vi "ENA_statuses.vi"(8 "error in (no error)":errorcluster caption="错误输入（无错误）", 11 "MotorSystem 输入":refnum<class "MotorSystem.lvclass">) -> (0 "error out":errorcluster caption="错误输出", 2 "ENA statuses":bool[](array[boolean]), 3 "MotorSystem 输出":refnum<class "MotorSystem.lvclass">)   [LabVIEW 2016, in "MotionControl_UFO_3DOF.lvlib" / "MotorSystem.lvclass"]
uses:
  <userlib>/MotionControl_UFO_3DOF/MotorSystem/MotorSystem.lvclass
  <userlib>/MotionControl_UFO_3DOF/MotorSystem/MotorSystem.lvclass/MotorSystem.ctl
  <userlib>/MotionControl_UFO_3DOF/OneMotion/OneMotion.lvclass/OneMotion.ctl
  <userlib>/MotionControl_UFO_3DOF/StepMotor/StepMotor.lvclass
  <userlib>/MotionControl_UFO_3DOF/OneMotion/OneMotion.lvclass
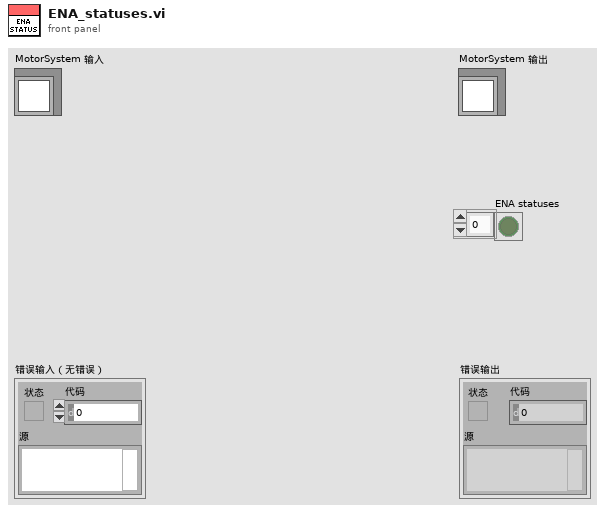
[diagram p1: front panel]
types:
  T1 = typedef "MotionControl_UFO_3DOF.lvlib/MotorSystem.lvclass/MotionCluster.ctl" = cluster{"OneMotion.lvclass":refnum<class "OneMotion.lvclass">, "connected?":bool, "default enabled?":bool, "enabled?":bool}
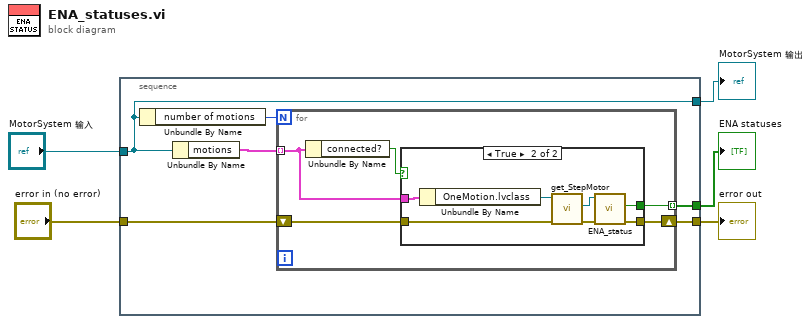
[diagram p0: block diagram]
diagram:
  n1 = stacked-sequence {
    tunnel: [w6] -> w5
    tunnel: [w11] -> w3
    tunnel: "MotorSystem 输入" -> [w11]
    tunnel: "error in (no error)" -> [w7]
    tunnel: [w8] -> w1
    frame #0 {
      n2 = Unbundle By Name(w11) -> ("number of motions"=w10:i32)
      n3 = Unbundle By Name(w11) -> ("motions"=w9:T1[])
      n4 = for {
        N: w10 -> [_]
        tunnel: w9 -> [w13] mode=indexing
        tunnel: [w16] -> w8 mode=indexing
        shift-right: [w14] -> w6
        shift-left: w7 -> [w15]
        n5 = Unbundle By Name(w13) -> ("connected?"=w12:bool)
        n6 = case shown="True" w12 {
          tunnel: w13 -> [_ w24]
          tunnel: [_ w21] -> w16
          tunnel: w15 -> [w17 w20]
          tunnel: [w17 w18] -> w14
          frame False {
          }
          frame True {
            n7 = Unbundle By Name(w24) -> ("OneMotion.lvclass"=w23:refnum<class "OneMotion.lvclass">)
            n8 = call <userlib>:"get_StepMotor.vi"("error in (no error)"=w20, "OneMotion输入"=w23) -> ("error out"=w19:errorcluster, "StepMotor.lvclass"=w22:refnum<class "StepMotor.lvclass">)  [unwired: 7 in, 1 out]
            n9 = call <userlib>:"ENA_status.vi"("error in (no error)"=w19, "StepMotor 输入"=w22) -> ("error out"=w18:errorcluster, "ENA status"=w21:bool)  [unwired: 7 in, 1 out]
          }
        }
      }
    }
  }
  "error out" <- w5
  "MotorSystem 输出" <- w3
  "ENA statuses" <- w1
